vi "Main_SubVI_Sort Comment_2.vi"(8 "Error In":errorcluster, 9 "Datas":i32[](array[numeric]), 10 "Register  Address":i32, 11 "Axis Number":T1=1 items=["X"=1, "Y"=2, "Z"=3, "Rotation"=4]) -> (0 "Error Out":errorcluster, 3 "Command":string)   [LabVIEW 2015]
uses:
  Control/Control_Axis Number.ctl
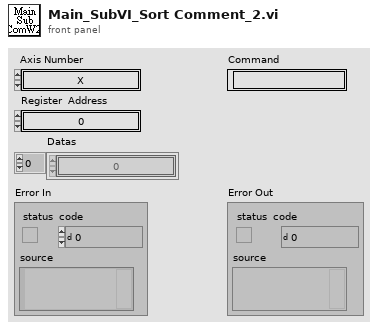
[diagram p1: front panel]
types:
  T1 = typedef "Control_Axis Number.ctl" = u16
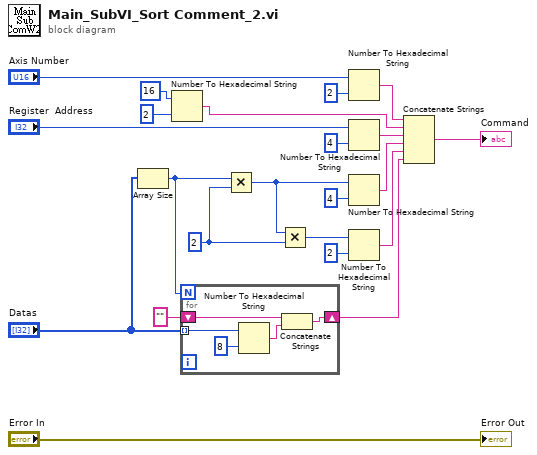
[diagram p0: block diagram]
diagram:
  w10 = 2 ("y")
  n1 = Array Size(array="Datas") -> (size(s)=w7:i32)
  n2 = Number To Hexadecimal String(1:i16 2 ("width (-)"), 2:16 ("number")) -> (0:w17:string)
  n3 = for {
    N: w7 -> [_]
    tunnel: "Datas" -> [w26] mode=indexing
    shift-right: [w25] -> w13
    shift-left: "" -> [w24]
    n4 = Number To Hexadecimal String(1:i16 8 ("width (-)"), 2:w26) -> (0:w23:string)
    n5 = Concatenate Strings(w24, w23) -> (w25:string)
  }
  n6 = Multiply(x=w7, y=w10) -> (x*y=w8:i32)
  n7 = Multiply(x=w8, y=w10) -> (x*y=w9:i32)
  n8 = Number To Hexadecimal String(1:i16 2 ("width (-)"), 2:"Axis Number") -> (0:w6:string)
  n9 = Number To Hexadecimal String(1:i16 4 ("width (-)"), 2:"Register  Address") -> (0:w16:string)
  n10 = Number To Hexadecimal String(1:i16 4 ("width (-)"), 2:w8) -> (0:w11:string)
  n11 = Number To Hexadecimal String(1:i16 2 ("width (-)"), 2:w9) -> (0:w12:string)
  n12 = Concatenate Strings(w6, w17, w16, w11, w12, w13) -> (→"Command":string)
  "Error Out" <- "Error In"
